vi "cDAQ Scale 4-20 sig.vi"(0 "4 mA y- value":dbl, 5 "20 mA y-value":dbl, 7 "Drop resistor":dbl) -> (4 "M":dbl, 6 "B":dbl)   [LabVIEW 2014]
doc: "Converts analog voltage to physical measurement. Use for the 4-20 mA current sensors."
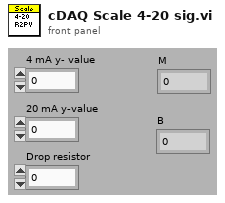
[diagram p1: front panel]
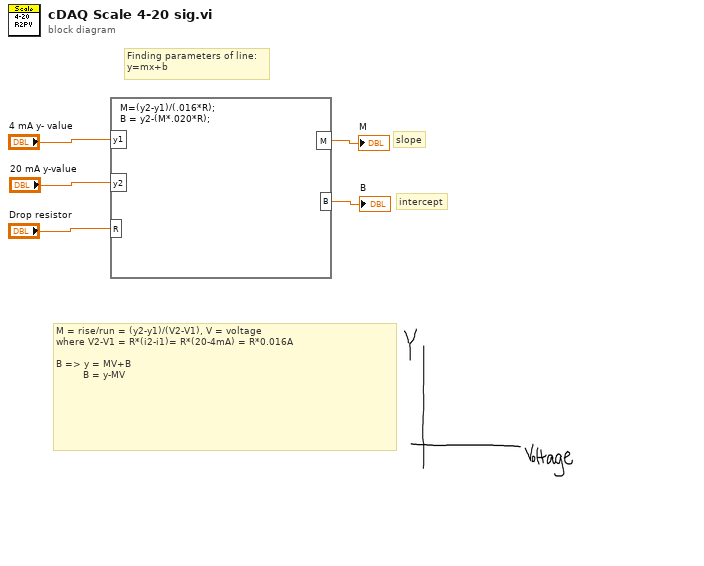
[diagram p0: block diagram]
diagram:
  # "M = rise/run = (y2-y1)/(V2-V1), V = voltage\nwhere V2-V1 = R*(i2-i1)= R*(20-4mA) = R*0.016A\n\nB => y = MV+B\n         B = y-MV"
  # "intercept"
  # "slope"
  # "Finding parameters of line:\ny=mx+b"
  n1 = formula code="M=(y2-y1)/(.016*R);\nB = y2-(M*.020*R);"("y1"="4 mA y- value", "y2"="20 mA y-value", "R"="Drop resistor") -> ("M"=→"M":dbl, "B"=→"B":dbl)
